vi "XYVoltageFGV.vi"(0 "X Voltage":dbl min=-2.5 max=2.5 step=0.01 format="%.2g", 1 "Y Voltage":dbl min=-2.5 max=2.5 step=0.01 format="%.2g", 3 "Ring":T1 items=["Get", "Set X", "Set Y", "Set XY", "Internal"]) -> (7 "X Voltage 2":dbl, 8 "Y Voltage 2":dbl, 10 "Ring 2":T1 items=["Get", "Set X", "Set Y", "Set XY", "Internal"])   [LabVIEW 2013]
uses:
  Controls/XYVoltageFGV.ctl
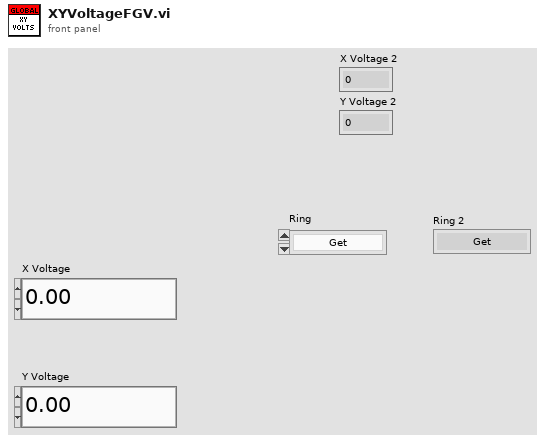
[diagram p1: front panel]
types:
  T1 = typedef "XYVoltageFGV.ctl" = u16
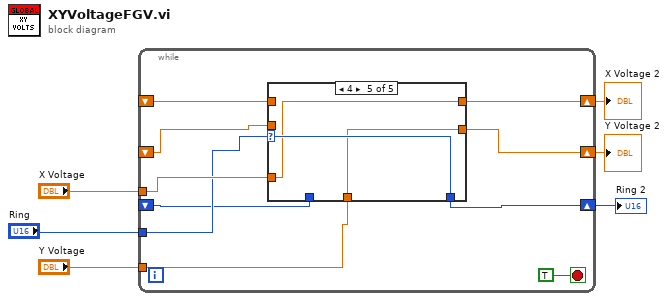
[diagram p0: block diagram]
diagram:
  n1 = while {
    shift-right: [w14] -> w4
    shift-left: _ -> [w15]
    shift-right: [w12] -> w3
    shift-left: _ -> [w13]
    tunnel: "X Voltage" -> [w11]
    tunnel: "Y Voltage" -> [w10]
    shift-right: [w8] -> w2
    shift-left: _ -> [w7]
    tunnel: "Ring" -> [w9]
    stop <- TRUE stop-if-true
    n2 = case shown="4" w9 {
      selector: w9 -> [_ w20 w23 w26 w31]
      tunnel: [w19 w22 w24 w28 w30] -> w14
      tunnel: w15 -> [w19 _ w24 _ _]
      tunnel: [w18 w21 w25 w27 w29] -> w12
      tunnel: w13 -> [w18 w21 _ _ _]
      tunnel: w11 -> [_ w22 _ w28 w30]
      tunnel: w10 -> [_ _ w25 w27 w29]
      tunnel: [w17 w20 w23 w26 w31] -> w8
      tunnel: w7 -> [w17 _ _ _ _]
      frame 0, Default {
      }
      frame 1 {
      }
      frame 2 {
      }
      frame 3 {
      }
      frame 4 {
      }
    }
  }
  "X Voltage 2" <- w4
  "Y Voltage 2" <- w3
  "Ring 2" <- w2
